vi "FIB HV & LEAKAGE MONITOR.vi"() -> ()   [LabVIEW 2018]
uses:
  <vilib>/DAQmx/write.llb/DAQmx Write (Analog 1D DBL NChan 1Samp).vi
  <vilib>/Analysis/baseanly.llb/Mean (DBL).vi
  <vilib>/DAQmx/read.llb/DAQmx Read (Analog 1D DBL NChan 1Samp).vi
  <vilib>/DAQmx/miscellaneous.llb/DAQmx Fill In Error Info.vi
  <vilib>/Analysis/NI_AALBase.lvlib
panel:
  out "COLUMN STARCELL":dbl format="%#_6p"
  out "ION SOURCE STARCELL":dbl format="%#_6p"
  in  "data":dbl[](array[numeric])
  out "ENERGY CONTROL":dbl
  out "Waveform Chart 3":dbl[](graph)
  out "Waveform Chart 2":dbl[](graph)
  out "Waveform Chart":dbl[](graph)
  in  "stop":bool
  out "ENERGY LEAKAGE":dbl
  out "ENERGY MON":dbl
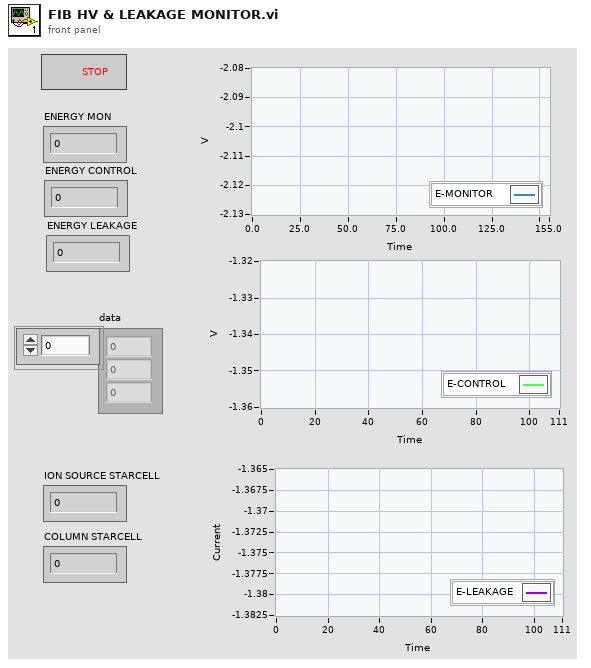
[diagram p1: front panel]
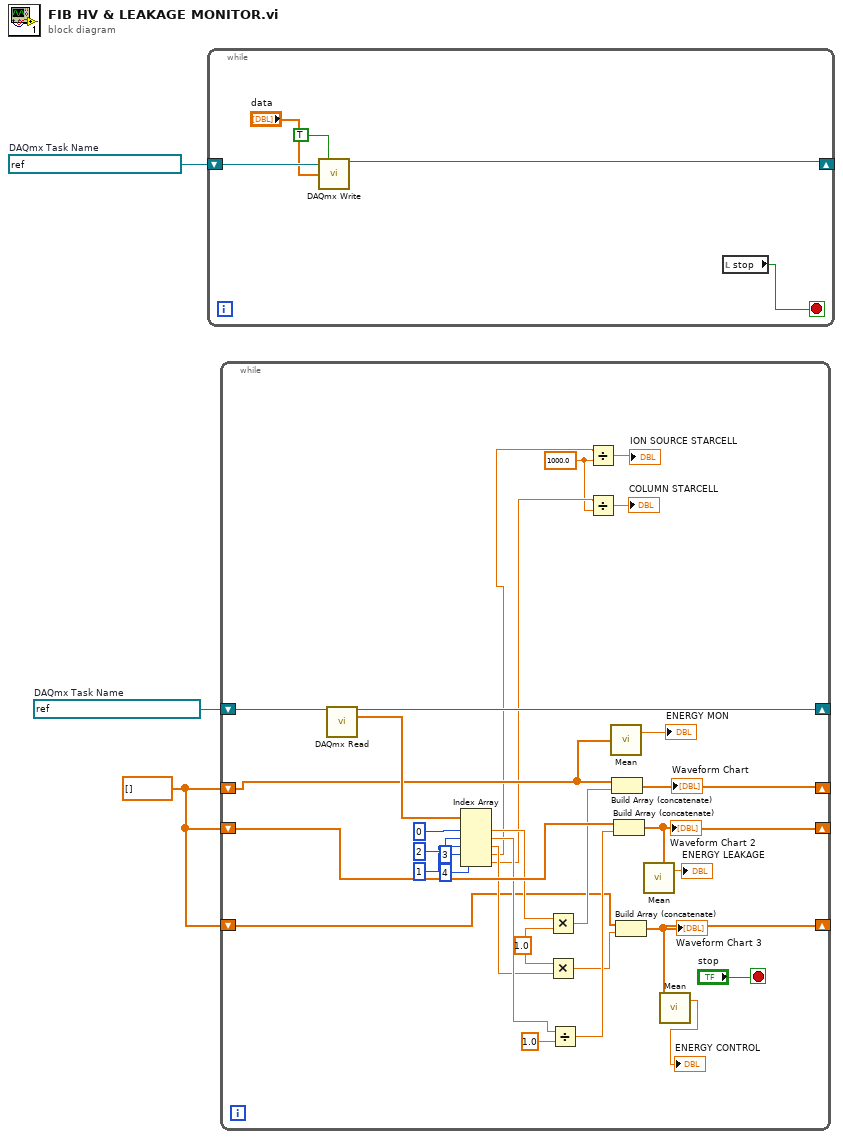
[diagram p0: block diagram]
diagram:
  w1 = refnum<k21> "FIB ION SOURCE CONTROL"  # DAQmx Task Name
  w2 = dbl[] []
  w3 = refnum<k21> "HV MONITOR & LEAKAGE"  # DAQmx Task Name
  n1 = while {
    shift-right: [w6] -> _
    shift-left: w1 -> [w8]
    stop <- w4 stop-if-true
    n2 = call-poly <vilib>:"DAQmx Write.vi"("task/channels in"=w8, "auto start"=TRUE, "data"="data") -> ("task out"=w6:refnum<k21>)  [unwired: 10 in, 2 out]
    n3 = local read "stop"() -> (w4:bool)
  }
  n4 = while {
    shift-right: [w38] -> _
    shift-left: w3 -> [w39]
    shift-right: [w33] -> _
    shift-left: w2 -> [w29]
    shift-right: [w24] -> _
    shift-left: w2 -> [w32]
    shift-right: [w17] -> _
    shift-left: w2 -> [w19]
    stop <- "stop" stop-if-true
    w11 = 1000.0 ("y")
    w21 = 1.0 ("x")
    n5 = call-poly <vilib>:"DAQmx Read.vi"("task/channels in"=w39) -> ("task out"=w38:refnum<k21>, "data"=w36:dbl[])  [unwired: 12 in, 1 out]
    n6 = Index Array(array=w36, index #1=0 ("index"), index #2=2 ("index"), index #3=1 ("index"), index #4=3 ("index"), index #5=4 ("index")) -> (element #1=w31:dbl, element #2=w26:dbl, element #3=w20:dbl, element #4=w13:dbl, element #5=w12:dbl)
    n7 = Multiply(x=w31, y=w21) -> (x*y=w30:dbl)
    n8 = Multiply(x=w21, y=w20) -> (x*y=w18:dbl)
    n9 = Divide(x=w26, y=1.0) -> (x/y=w25:dbl)
    n10 = Divide(x=w13, y=w11) -> (x/y=→"ION SOURCE STARCELL":dbl)
    n11 = Divide(x=w12, y=w11) -> (x/y=→"COLUMN STARCELL":dbl)
    n12 = call-poly <vilib>:"Mean.vi"("X"=w29) -> ("mean"=→"ENERGY MON":dbl)  [unwired: 1 out]
    n13 = Build Array (concatenate)(w29, w30) -> (w33:dbl[])
    "Waveform Chart" <- w33
    n14 = Build Array (concatenate)(w32, w25) -> (w24:dbl[])
    "Waveform Chart 2" <- w24
    n15 = Build Array (concatenate)(w19, w18) -> (w17:dbl[])
    "Waveform Chart 3" <- w17
    n16 = call-poly <vilib>:"Mean.vi"("X"=w24) -> ("mean"=→"ENERGY LEAKAGE":dbl)  [unwired: 1 out]
    n17 = call-poly <vilib>:"Mean.vi"("X"=w17) -> ("mean"=→"ENERGY CONTROL":dbl)  [unwired: 1 out]
  }
